vi "VI Tree.vi"   [LabVIEW 2009, in "Digikrom DK24x.lvlib"]
doc: "This is the instrument driver for the <INSTRUMENT NAME>. The VI Tree displays all the user-callable VIs of the instrument driver in an organized table."
uses:
  Digikrom DK24x.lvlib
  Utility/Calibration/Calibrate Slit (1).vi
  Configure/Adjust Slit (1).vi
  Action-Status/Scan (Up).vi
panel:
  # "(c) 2007 <Enter Company Name Here>.  ALL RIGHTS RESERVED."
  # "SEE DIAGRAM\nFOR VI TREE."
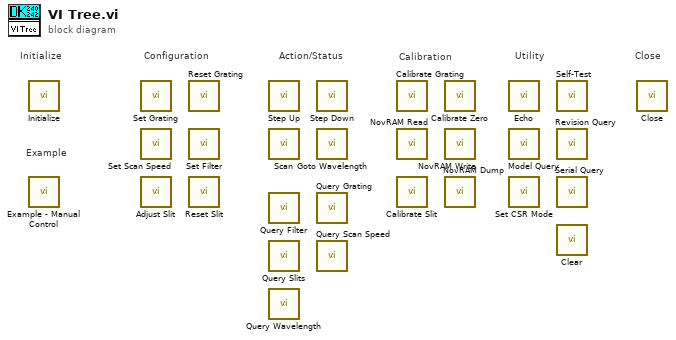
[diagram p0: block diagram]
diagram:
  # "Calibration"
  # "Example"
  # "Configuration"
  # "Utility"
  # "Action/Status"
  # "Close"
  # "Initialize"
  n1 = call "Initialize.vi"() -> ()  [unwired: 10 in, 2 out]
  n2 = call "Example - Manual Control.vi"() -> ()  [unwired: 2 in]
  n3 = call "Set Grating.vi"() -> ()  [unwired: 10 in, 2 out]
  n4 = call "Set Scan Speed.vi"() -> ()  [unwired: 10 in, 2 out]
  n5 = call-poly "Adjust Slit.vi"() -> ()  [unwired: 10 in, 2 out]
  n6 = call "Reset Grating.vi"() -> ()  [unwired: 10 in, 2 out]
  n7 = call "Set Filter.vi"() -> ()  [unwired: 10 in, 2 out]
  n8 = call "Reset Slit.vi"() -> ()  [unwired: 10 in, 2 out]
  n9 = call "Step Up.vi"() -> ()  [unwired: 10 in, 2 out]
  n10 = call-poly "Scan.vi"() -> ()  [unwired: 10 in, 2 out]
  n11 = call "Query Filter.vi"() -> ()  [unwired: 9 in, 3 out]
  n12 = call "Query Slits.vi"() -> ()  [unwired: 7 in, 5 out]
  n13 = call "Query Wavelength.vi"() -> ()  [unwired: 9 in, 3 out]
  n14 = call "Step Down.vi"() -> ()  [unwired: 8 in, 2 out]
  n15 = call "Goto Wavelength.vi"() -> ()  [unwired: 10 in, 2 out]
  n16 = call "Query Grating.vi"() -> ()  [unwired: 6 in, 6 out]
  n17 = call "Query Scan Speed.vi"() -> ()  [unwired: 9 in, 3 out]
  n18 = call "Calibrate Grating.vi"() -> ()  [unwired: 10 in, 2 out]
  n19 = call "NovRAM Read.vi"() -> ()  [unwired: 9 in, 3 out]
  n20 = call-poly "Calibrate Slit.vi"() -> ()  [unwired: 10 in, 2 out]
  n21 = call "Calibrate Zero.vi"() -> ()  [unwired: 10 in, 2 out]
  n22 = call "NovRAM Write.vi"() -> ()  [unwired: 10 in, 2 out]
  n23 = call "NovRAM Dump.vi"() -> ()  [unwired: 12 in]
  n24 = call "Echo.vi"() -> ()  [unwired: 9 in, 3 out]
  n25 = call "Model Query.vi"() -> ()  [unwired: 9 in, 3 out]
  n26 = call "Set CSR Mode.vi"() -> ()  [unwired: 9 in, 3 out]
  n27 = call "Self-Test.vi"() -> ()  [unwired: 9 in, 3 out]
  n28 = call "Revision Query.vi"() -> ()  [unwired: 8 in, 4 out]
  n29 = call "Serial Query.vi"() -> ()  [unwired: 9 in, 3 out]
  n30 = call "Clear.vi"() -> ()  [unwired: 10 in, 2 out]
  n31 = call "Close.vi"() -> ()  [unwired: 11 in, 1 out]
